vi "Dance.vi"() -> ()   [LabVIEW 2016]
uses:
  AerotechLibraries/Motion/EnableMultiple.vi
panel:
  in  "Stop Button":bool
  # "XYZ Stage Dance!!! Brookhaven National Laboratory"
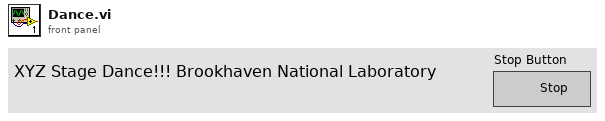
[diagram p1: front panel]
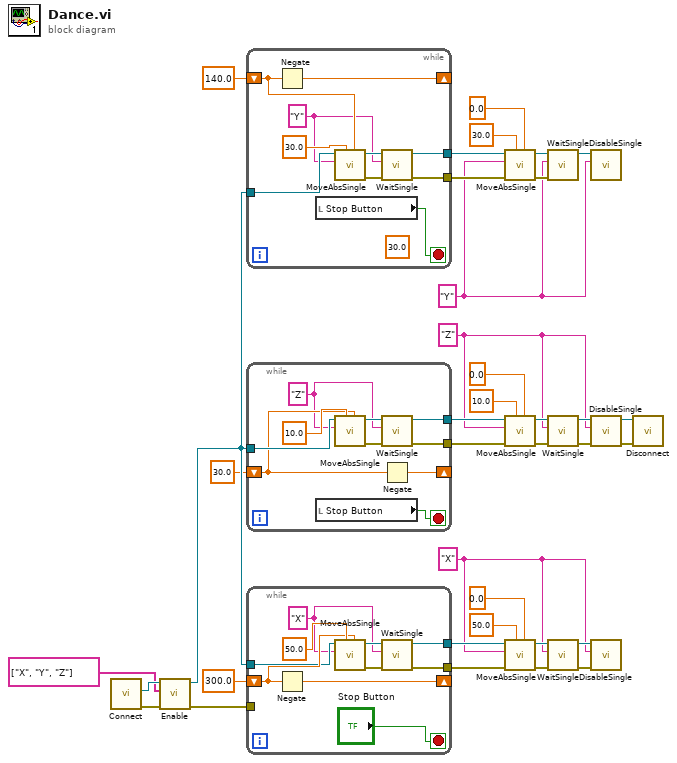
[diagram p0: block diagram]
diagram:
  w3 = "X" ("axis name")
  w13 = "Z" ("axis name")
  w17 = "Y" ("axis name")
  n1 = call "Connect.vi"() -> ("error out"=w34:errorcluster, "controller"=w36:refnum<k24>)  [unwired: 10 in]
  n2 = call-poly "Enable.vi"("error in (no error)"=w34, "axis names"=string[] ["X", "Y", "Z"], "controller in"=w36) -> ("error out"=w33:errorcluster, "controller out"=w31:refnum<k24>)  [unwired: 7 in]
  n3 = while {
    tunnel: w31 -> [w43]
    shift-right: [w42] -> _
    shift-left: 140.0 -> [w41]
    tunnel: [w38] -> w28
    tunnel: [w37] -> w27
    stop <- w46 stop-if-true
    (unwired) 30.0 ("speed")
    w39 = "Y" ("axis name")
    n4 = Negate(x=w41) -> (-x=w42:dbl)
    n5 = local read "Stop Button"() -> (w46:bool)
    n6 = call "MoveAbsSingle.vi"("position"=w41, "speed"=30.0, "axis name"=w39, "controller in"=w43) -> ("error out"=w44:errorcluster, "controller out"=w45:refnum<k24>)  [unwired: 6 in]
    n7 = call "WaitSingle.vi"("error in (no error)"=w44, "axis name"=w39, "controller in"=w45) -> ("error out"=w37:errorcluster, "controller out"=w38:refnum<k24>)  [unwired: 6 in, 1 out]
  }
  n8 = while {
    tunnel: w31 -> [w54]
    shift-right: [w53] -> _
    shift-left: 30.0 -> [w52]
    tunnel: [w48] -> w24
    tunnel: [w47] -> w21
    stop <- w56 stop-if-true
    w49 = "Z" ("axis name")
    n9 = local read "Stop Button"() -> (w56:bool)
    n10 = call "MoveAbsSingle.vi"("position"=w52, "speed"=10.0, "axis name"=w49, "controller in"=w54) -> ("error out"=w50:errorcluster, "controller out"=w51:refnum<k24>)  [unwired: 6 in]
    n11 = call "WaitSingle.vi"("error in (no error)"=w50, "axis name"=w49, "controller in"=w51) -> ("error out"=w47:errorcluster, "controller out"=w48:refnum<k24>)  [unwired: 6 in, 1 out]
    n12 = Negate(x=w52) -> (-x=w53:dbl)
  }
  n13 = while {
    tunnel: w33 -> [_]
    tunnel: w31 -> [w63]
    shift-right: [w65] -> _
    shift-left: 300.0 -> [w64]
    tunnel: [w60] -> w8
    tunnel: [w57] -> w9
    stop <- "Stop Button" stop-if-true
    w59 = "X" ("axis name")
    n14 = Negate(x=w64) -> (-x=w65:dbl)
    n15 = call "MoveAbsSingle.vi"("position"=w64, "speed"=50.0, "axis name"=w59, "controller in"=w63) -> ("error out"=w58:errorcluster, "controller out"=w61:refnum<k24>)  [unwired: 6 in]
    n16 = call "WaitSingle.vi"("error in (no error)"=w58, "axis name"=w59, "controller in"=w61) -> ("error out"=w57:errorcluster, "controller out"=w60:refnum<k24>)  [unwired: 6 in, 1 out]
  }
  n17 = call "MoveAbsSingle.vi"("position"=0.0, "speed"=30.0, "error in (no error)"=w27, "axis name"=w17, "controller in"=w28) -> ("error out"=w19:errorcluster, "controller out"=w20:refnum<k24>)  [unwired: 5 in]
  n18 = call "MoveAbsSingle.vi"("position"=0.0, "speed"=10.0, "error in (no error)"=w21, "axis name"=w13, "controller in"=w24) -> ("error out"=w16:errorcluster, "controller out"=w15:refnum<k24>)  [unwired: 5 in]
  n19 = call "MoveAbsSingle.vi"("position"=0.0, "speed"=50.0, "error in (no error)"=w9, "axis name"=w3, "controller in"=w8) -> ("error out"=w6:errorcluster, "controller out"=w7:refnum<k24>)  [unwired: 5 in]
  n20 = call "WaitSingle.vi"("error in (no error)"=w19, "axis name"=w17, "controller in"=w20) -> ("controller out"=w18:refnum<k24>)  [unwired: 6 in, 2 out]
  n21 = call "WaitSingle.vi"("error in (no error)"=w16, "axis name"=w13, "controller in"=w15) -> ("error out"=w12:errorcluster, "controller out"=w14:refnum<k24>)  [unwired: 6 in, 1 out]
  n22 = call "WaitSingle.vi"("error in (no error)"=w6, "axis name"=w3, "controller in"=w7) -> ("error out"=w5:errorcluster, "controller out"=w4:refnum<k24>)  [unwired: 6 in, 1 out]
  n23 = call "DisableSingle.vi"("axis name"=w17, "controller in"=w18) -> ()  [unwired: 8 in, 2 out]
  n24 = call "DisableSingle.vi"("error in (no error)"=w12, "axis name"=w13, "controller in"=w14) -> ("error out"=w10:errorcluster, "controller out"=w11:refnum<k24>)  [unwired: 7 in]
  n25 = call "DisableSingle.vi"("error in (no error)"=w5, "axis name"=w3, "controller in"=w4) -> ()  [unwired: 7 in, 2 out]
  n26 = call "Disconnect.vi"("error in (no error)"=w10, "controller"=w11) -> ()  [unwired: 9 in, 1 out]
